vi "Get Instrument Alias.vi"(8 "error in (no error)":errorcluster, 11 "SDS1104X-E in":refnum<class "SDS1104X-E.lvclass">) -> (0 "error out":errorcluster, 2 "Instrument Alias":string, 3 "SDS1104X-E out":refnum<class "SDS1104X-E.lvclass">)   [LabVIEW 2023, in "HAF.lvlib" / "SDS1104X-E.lvclass"]
doc: "Returns the alias name of the Instrument for this Driver that can be used to initiate a session. Must be implemented by Subclasses because there is no Visa Session available to obtain it from when it is needed.\n\nIt's not ideal: need to think of a better way of dealing with attached resources than hard-coded aliases which must match what was entered in NI-MAX."
uses:
  SDS1104X-E.lvclass
  SDS1104X-E.lvclass/SDS1104X-E.ctl
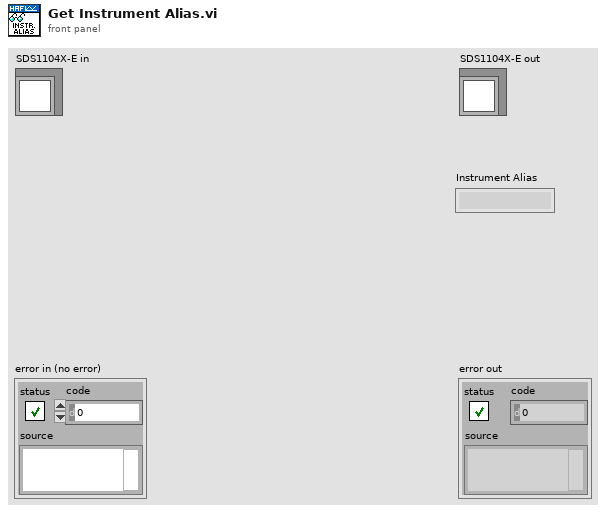
[diagram p1: front panel]
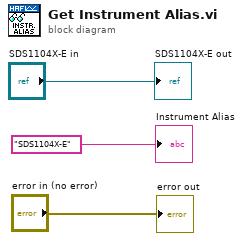
[diagram p0: block diagram]
diagram:
  "error out" <- "error in (no error)"
  "SDS1104X-E out" <- "SDS1104X-E in"
  "Instrument Alias" <- "SDS1104X-E" ("Instrument Alias")
